vi "solar_voy Read Voyager ID Offset.vi"(8 "error in (no error)":errorcluster, 11 "Config Path in":path) -> (0 "error out":errorcluster, 3 "VoyagerIDOffset":u16)   [LabVIEW 2018]
doc: "Read Voyager ID Offset from file. The values will default to 10000, and then 1000 more for each target."
uses:
  cfg/solar_cfg Read File (Str).vi
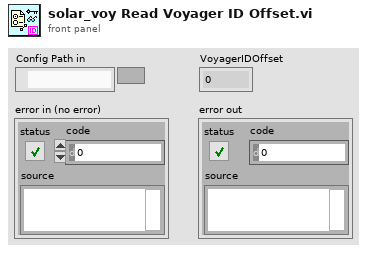
[diagram p1: front panel]
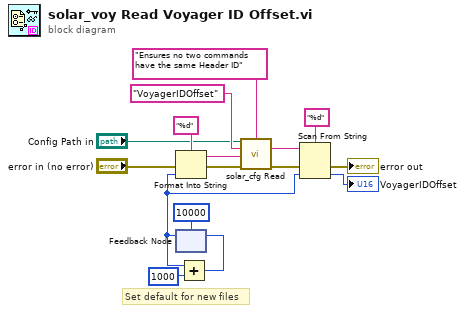
[diagram p0: block diagram]
diagram:
  # "Set default for new files"
  n1 = feedback #1(u16 10000) -> (w15:u16)
  n2 = Format Into String(format string="%d", error in="error in (no error)", w15) -> (resulting string=w9:string, error out=w7:errorcluster)  [unwired: 1 in]
  n3 = Add(x=w15, y=u16 1000) -> (x+y=w5:u16)
  n4 = feedback-in #1(w5) -> ()
  n5 = call-poly "solar_cfg Read.vi"("Config Path (*.ini)"="Config Path in", "Comment"="Ensures no two commands have the same Header ID", "Key"="VoyagerIDOffset", "Value in"=w9, "error in (no error)"=w7) -> ("Value out"=w13:string, "error out"=w11:errorcluster)  [unwired: 7 in, 2 out]
  n6 = Scan From String(format string="%d", input string=w13, error in=w11, default 1=w15) -> (error out=→"error out":errorcluster, output 1=→"VoyagerIDOffset":u16)  [unwired: 1 in, 2 out]
